vi "subVI_CONEX_absMove.vi"(3 "Error IN":errorcluster, 4 "Target Pos.":dbl[](array[numeric])=[0.0, 0.0, 0.0], 5 "CONEX Cluster":T1) -> (0 "error out":errorcluster, 2 "CONEX Cluster out":T1)   [LabVIEW 2010]
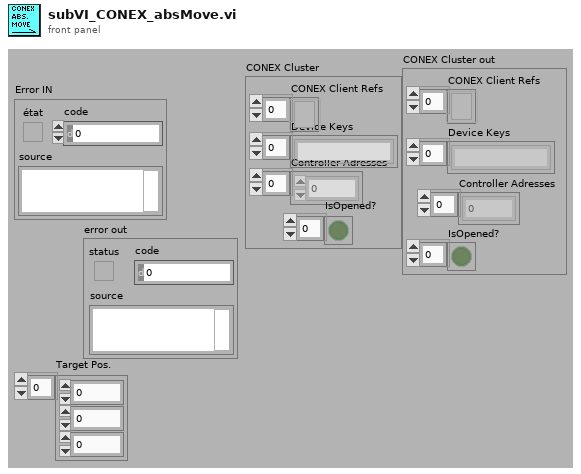
[diagram p1: front panel]
types:
  T1 = cluster{"CONEX Client Refs":refnum<k24>[], "Device Keys":string[], "Controller Adresses":i32[], "IsOpened?":bool[]}
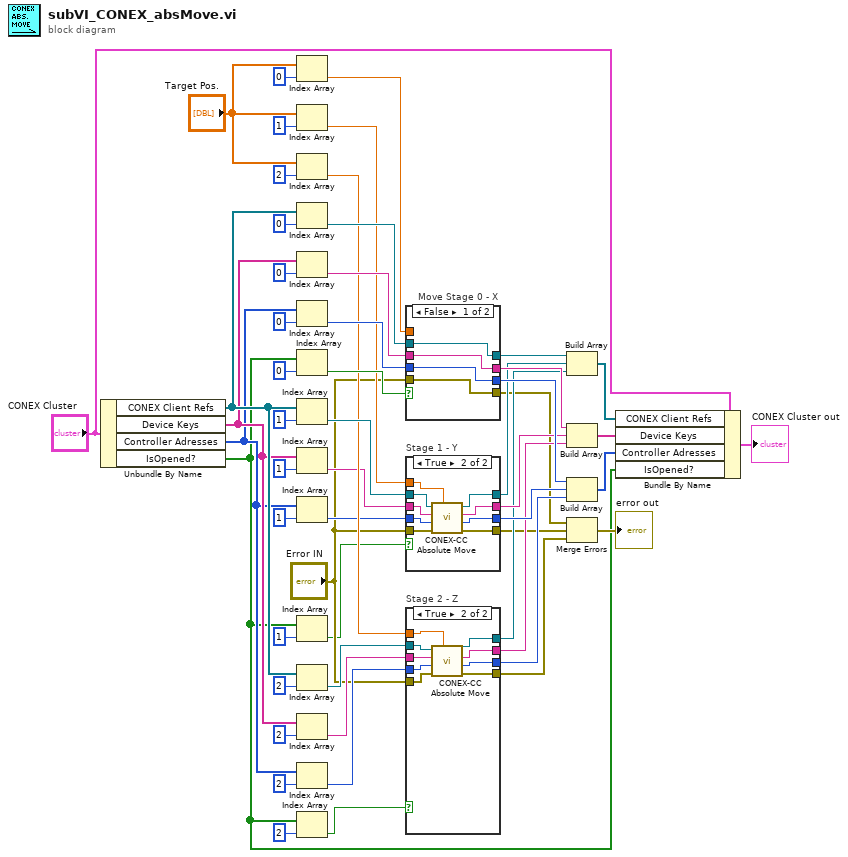
[diagram p0: block diagram]
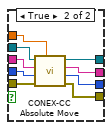
[diagram p4: hidden frame]
diagram:
  n1 = Unbundle By Name("CONEX Cluster") -> ("CONEX Client Refs"=w51:refnum<k24>[], "Device Keys"=w46:string[], "Controller Adresses"=w41:i32[], "IsOpened?"=w3:bool[])
  n2 = Index Array(array="Target Pos.", index=0) -> (element=w29:dbl)
  n3 = Index Array(array="Target Pos.", index=1) -> (element=w24:dbl)
  n4 = Index Array(array="Target Pos.", index=2) -> (element=w21:dbl)
  n5 = Index Array(array=w51, index=0) -> (element=w50:refnum<k24>)
  n6 = Index Array(array=w46, index=0) -> (element=w45:string)
  n7 = Index Array(array=w41, index=0) -> (element=w40:i32)
  n8 = Index Array(array=w3, index=0) -> (element=w26:bool)
  n9 = Index Array(array=w51, index=1) -> (element=w23:refnum<k24>)
  n10 = Index Array(array=w46, index=1) -> (element=w20:string)
  n11 = Index Array(array=w41, index=1) -> (element=w17:i32)
  n12 = Index Array(array=w3, index=1) -> (element=w1:bool)
  n13 = Index Array(array=w51, index=2) -> (element=w22:refnum<k24>)
  n14 = Index Array(array=w46, index=2) -> (element=w19:string)
  n15 = Index Array(array=w41, index=2) -> (element=w18:i32)
  n16 = Index Array(array=w3, index=2) -> (element=w4:bool)
  n17 = case "Move Stage 0 - X" shown="False" w26 {
    tunnel: w50 -> [w55 w67]
    tunnel: w45 -> [w56 w66]
    tunnel: w40 -> [w57 w65]
    tunnel: "Error IN" -> [w58 w64]
    tunnel: [w55 w63] -> w39
    tunnel: [w56 w62] -> w38
    tunnel: [w57 w61] -> w37
    tunnel: w29 -> [_ w60]
    tunnel: [w58 w59] -> w6
    frame False {
    }
    frame True {
      n18 = call <userlib>:"CONEX-CC Absolute Move.vi"("Target position"=w60, "Error IN"=w64, "Address IN"=w65, "deviceKey IN"=w66, "CONEX Client Ref IN"=w67) -> ("Error OUT"=w59:errorcluster, "Address OUT"=w61:i32, "deviceKey OUT"=w62:string, "CONEX Client Ref OUT"=w63:refnum<k24>)  [unwired: 1 in]
    }
  }
  n19 = case "Stage 1 - Y" shown="True" w1 {
    tunnel: w23 -> [w68 w80]
    tunnel: w20 -> [w69 w79]
    tunnel: w17 -> [w70 w78]
    tunnel: "Error IN" -> [w71 w77]
    tunnel: [w68 w76] -> w10
    tunnel: [w69 w75] -> w13
    tunnel: [w70 w74] -> w14
    tunnel: w24 -> [_ w73]
    tunnel: [w71 w72] -> w9
    frame False {
    }
    frame True {
      n20 = call <userlib>:"CONEX-CC Absolute Move.vi"("Target position"=w73, "Error IN"=w77, "Address IN"=w78, "deviceKey IN"=w79, "CONEX Client Ref IN"=w80) -> ("Error OUT"=w72:errorcluster, "Address OUT"=w74:i32, "deviceKey OUT"=w75:string, "CONEX Client Ref OUT"=w76:refnum<k24>)  [unwired: 1 in]
    }
  }
  n21 = case "Stage 2 - Z" shown="True" w4 {
    tunnel: w22 -> [w81 w93]
    tunnel: w19 -> [w82 w92]
    tunnel: w18 -> [w83 w91]
    tunnel: "Error IN" -> [w84 w90]
    tunnel: [w81 w89] -> w11
    tunnel: [w82 w88] -> w12
    tunnel: [w83 w87] -> w15
    tunnel: w21 -> [_ w86]
    tunnel: [w84 w85] -> w8
    frame False {
    }
    frame True {
      n22 = call <userlib>:"CONEX-CC Absolute Move.vi"("Target position"=w86, "Error IN"=w90, "Address IN"=w91, "deviceKey IN"=w92, "CONEX Client Ref IN"=w93) -> ("Error OUT"=w85:errorcluster, "Address OUT"=w87:i32, "deviceKey OUT"=w88:string, "CONEX Client Ref OUT"=w89:refnum<k24>)  [unwired: 1 in]
    }
  }
  n23 = Build Array(w39, w10, w11) -> (w36:refnum<k24>[])
  n24 = Build Array(w38, w13, w12) -> (w35:string[])
  n25 = Build Array(w37, w14, w15) -> (w34:i32[])
  n26 = Merge Errors(w6, w9, w8) -> (→"error out":errorcluster)
  n27 = Bundle By Name(cluster="CONEX Cluster", "CONEX Client Refs"=w36, "Device Keys"=w35, "Controller Adresses"=w34, "IsOpened?"=w3) -> (→"CONEX Cluster out":T1)
